vi "mouse_ctrl init.vi"(8 "error in (no error)":errorcluster, 10 "refnum cluster input":T1, 11 "mouse_ctrl in":refnum<class "mouse_ctrl.lvclass">) -> (0 "error out":errorcluster, 3 "mouse_ctrl out":refnum<class "mouse_ctrl.lvclass">)   [LabVIEW 2018, in "mouse_ctrl.lvclass"]
uses:
  mouse_ctrl.lvclass
  mouse_ctrl.lvclass/mouse_ctrl.ctl
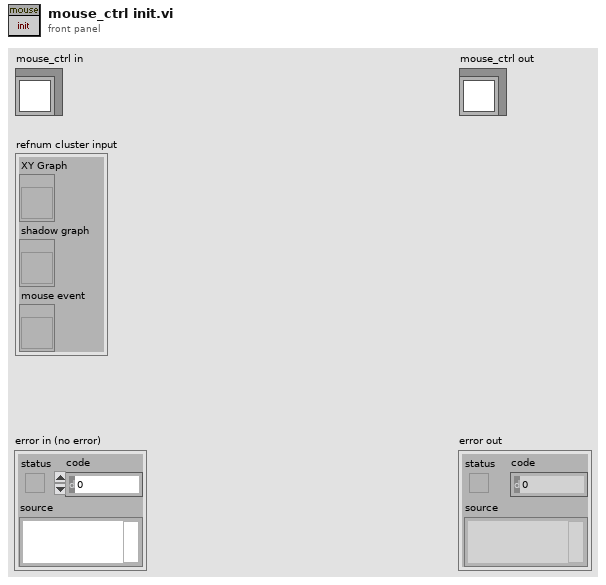
[diagram p1: front panel]
types:
  T1 = cluster{"XY Graph":refnum<vi>, "shadow graph":refnum<vi>, "mouse event":refnum<vi>}
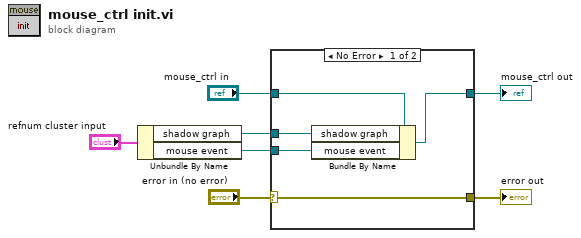
[diagram p0: block diagram]
diagram:
  n1 = Unbundle By Name("refnum cluster input") -> ("shadow graph"=w3:refnum<vi>, "mouse event"=w2:refnum<vi>)
  n2 = case shown="No Error" "error in (no error)" {
    selector: "error in (no error)" -> [w12 w14]
    tunnel: [w12 w14] -> w6
    tunnel: [w10 w13] -> w4
    tunnel: "mouse_ctrl in" -> [w11 w13]
    tunnel: w3 -> [w9 _]
    tunnel: w2 -> [w8 _]
    frame No Error {
      n3 = Bundle By Name(cluster=w11, "shadow graph"=w9, "mouse event"=w8) -> (w10:refnum<class "mouse_ctrl.lvclass">)
    }
    frame Error {
    }
  }
  "error out" <- w6
  "mouse_ctrl out" <- w4
